vi "ALTS-2015 LV2GBL INI Info.vi"(7 "Options":T2, 8 "error in":errorcluster, 11 "Configuration Cluster":T1={"Application"={"Rerun Count"=0, "Workorder No"="", "PLC Scanner"=FALSE, "Time Delay to Restart(mins)"=0.0}, "Station Details"={"Sensor Name 1"="", "Sensor Name 2"="", "Sensor Name 3"="", "Sensor Name 4"="", "Station1 Enable"=FALSE, "Station2 Enable"=FALSE, "Station3 Enable"=FALSE, "Station4 Enable"=FALSE}, "Database"={"Database Connection Link"=path "", "Result Procedure"="", "User"="", "Password"="", "Prompt"=FALSE, "Station 1 LT Result DB DSN Path"=path "", "Station 2 LT Result DB DSN Path"=path "", "Station 3 LT Result DB DSN Path"=path "", "Station 4 LT Result DB DSN Path"=path "", "AirLeakTestResult Procedure"="", "Serial Details Procedure"=""}, "Simulation"={"Simulate DAQ Hardware"=FALSE, "Simulate Result DB Write"=FALSE, "Simulate Scanner"=FALSE, "Simulate OPC"=FALSE, "Simulate Serial Details DB"=FALSE, "Simulate Result DB"=FALSE, "Simulate Scanner DB Path"=path "", "Simulate Serial Details DB Path"=path "", "Simulate Result DB Path"=path ""}, "Barcode Scanner1"={"Scanner IP"="", "Scanner Port"=0, "#Bytes to Read"=0, "Timeout_ms"=1000}, "Barcode Scanner2"={"Enabled?"=FALSE, "Scanner IP"="", "Scanner Port"=0, "#Bytes to Read"=0}}) -> (0 "error out":errorcluster, 3 "Configuration Cluster Out":T1={"Application"={"Rerun Count"=0, "Workorder No"="", "PLC Scanner"=FALSE, "Time Delay to Restart(mins)"=0.0}, "Station Details"={"Sensor Name 1"="", "Sensor Name 2"="", "Sensor Name 3"="", "Sensor Name 4"="", "Station1 Enable"=FALSE, "Station2 Enable"=FALSE, "Station3 Enable"=FALSE, "Station4 Enable"=FALSE}, "Database"={"Database Connection Link"=path "", "Result Procedure"="", "User"="", "Password"="", "Prompt"=FALSE, "Station 1 LT Result DB DSN Path"=path "", "Station 2 LT Result DB DSN Path"=path "", "Station 3 LT Result DB DSN Path"=path "", "Station 4 LT Result DB DSN Path"=path "", "AirLeakTestResult Procedure"="", "Serial Details Procedure"=""}, "Simulation"={"Simulate DAQ Hardware"=FALSE, "Simulate Result DB Write"=FALSE, "Simulate Scanner"=FALSE, "Simulate OPC"=FALSE, "Simulate Serial Details DB"=FALSE, "Simulate Result DB"=FALSE, "Simulate Scanner DB Path"=path "", "Simulate Serial Details DB Path"=path "", "Simulate Result DB Path"=path ""}, "Barcode Scanner1"={"Scanner IP"="", "Scanner Port"=0, "#Bytes to Read"=0, "Timeout_ms"=1000}, "Barcode Scanner2"={"Enabled?"=FALSE, "Scanner IP"="", "Scanner Port"=0, "#Bytes to Read"=0}})   [LabVIEW 2013]
uses:
  Controls/ALTS-2015 LV2GBL Options.ctl
  Controls/ALTS-2015 INI Configuration Cluster.ctl
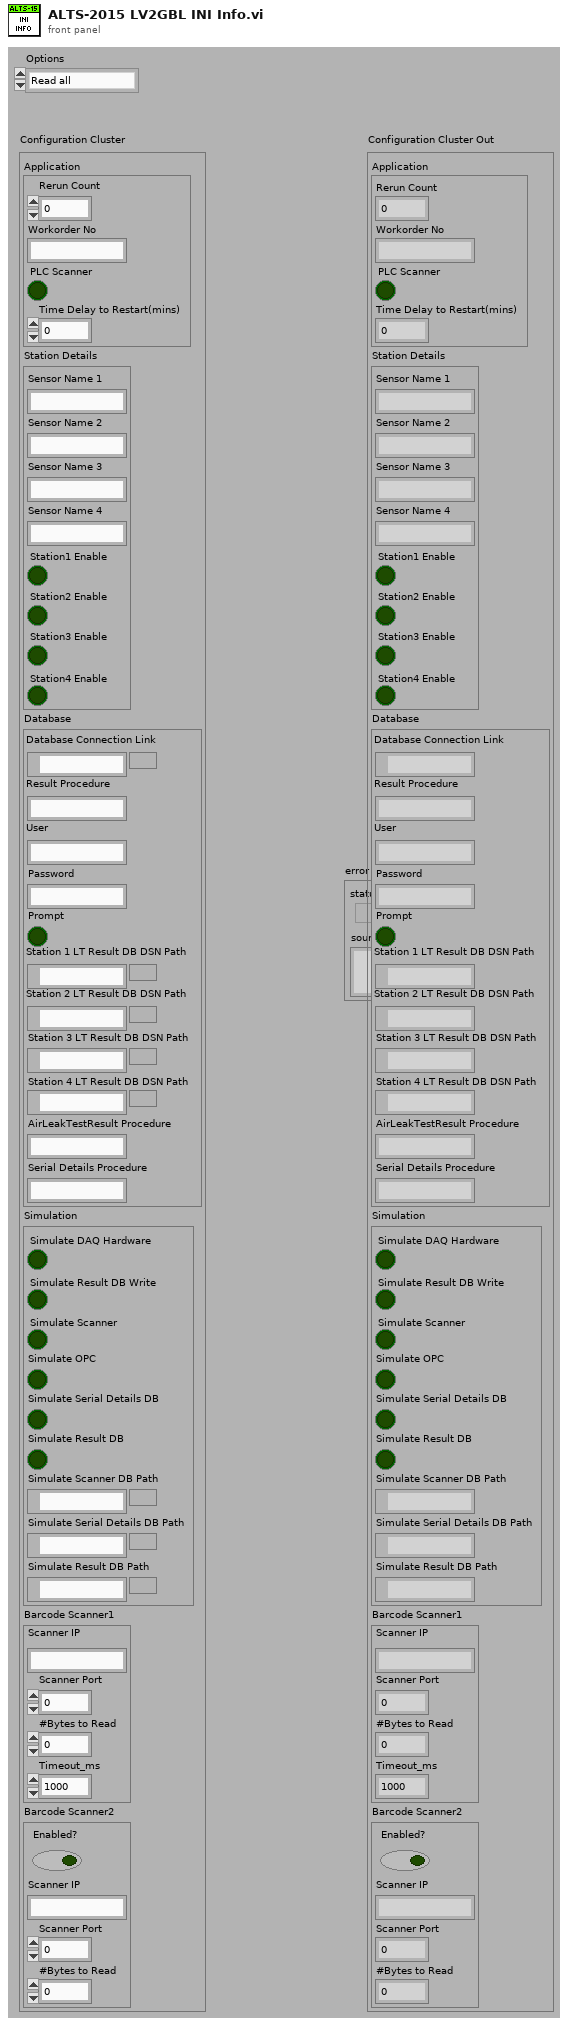
[diagram p1: front panel]
types:
  T1 = typedef "ALTS-2015 INI Configuration Cluster.ctl" = cluster{"Application":cluster{"Rerun Count":i32, "Workorder No":string, "PLC Scanner":bool, "Time Delay to Restart(mins)":dbl}, "Station Details":cluster{"Sensor Name 1":string, "Sensor Name 2":string, "Sensor Name 3":string, "Sensor Name 4":string, "Station1 Enable":bool, "Station2 Enable":bool, "Station3 Enable":bool, "Station4 Enable":bool}, "Database":cluster{"Database Connection Link":path, "Result Procedure":string, "User":string, "Password":string, "Prompt":bool, "Station 1 LT Result DB DSN Path":path, "Station 2 LT Result DB DSN Path":path, "Station 3 LT Result DB DSN Path":path, "Station 4 LT Result DB DSN Path":path, "AirLeakTestResult Procedure":string, "Serial Details Procedure":string}, "Simulation":cluster{"Simulate DAQ Hardware":bool, "Simulate Result DB Write":bool, "Simulate Scanner":bool, "Simulate OPC":bool, "Simulate Serial Details DB":bool, "Simulate Result DB":bool, "Simulate Scanner DB Path":path, "Simulate Serial Details DB Path":path, "Simulate Result DB Path":path}, "Barcode Scanner1":cluster{"Scanner IP":string, "Scanner Port":u16, "#Bytes to Read":i32, "Timeout_ms":i32}, "Barcode Scanner2":cluster{"Enabled?":bool, "Scanner IP":string, "Scanner Port":u16, "#Bytes to Read":i32}}
  T2 = typedef "ALTS-2015 LV2GBL Options.ctl" = enum16{"Read all", "Write all"}
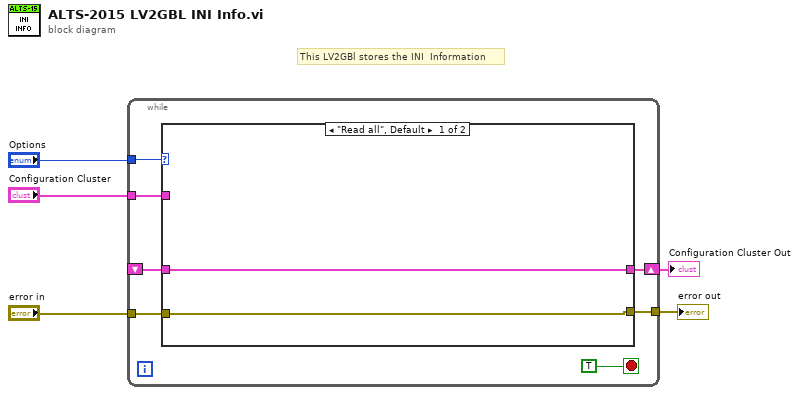
[diagram p0: block diagram]
diagram:
  # "This LV2GBl stores the INI  Information"
  n1 = while {
    shift-right: [w10] -> w1
    shift-left: _ -> [w11]
    tunnel: "Options" -> [w9]
    tunnel: "Configuration Cluster" -> [w8]
    tunnel: "error in" -> [w7]
    tunnel: [w6] -> w2
    stop <- TRUE stop-if-true
    n2 = case shown="\"Read all\", Default" w9 {
      tunnel: w11 -> [w14 _]
      tunnel: [w14 w16] -> w10
      tunnel: w8 -> [_ w16]
      tunnel: [w13 w15] -> w6
      tunnel: w7 -> [w13 w15]
      frame "Read all", Default {
      }
      frame "Write all" {
      }
    }
  }
  "error out" <- w2
  "Configuration Cluster Out" <- w1
